vi "Configure Report Generation.vi"(8 "error in (no error)":errorcluster, 9 "Report File Path":path, 10 "Report Type":string, 11 "Execution API In":refnum<class "Execution API.lvclass">) -> (0 "error out":errorcluster, 3 "Execution API Out":refnum<class "Execution API.lvclass">)   [LabVIEW 2020, in "Execution API.lvclass"]
uses:
  Execution API.lvclass
  Plugins/Report/Report.lvclass
  C:/git/astemes-lunit/source/Framework/Plugin/Plugin.lvclass
  Execution API.lvclass/Execution API.ctl
  Plugin Loader/Plugin Loader.lvclass
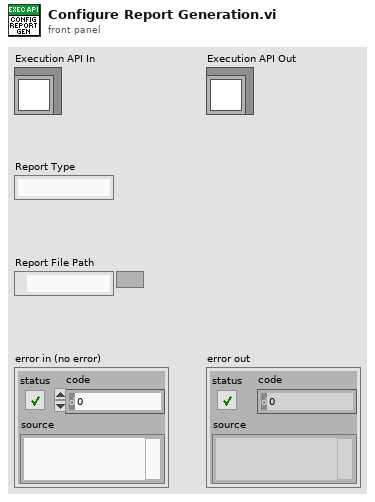
[diagram p1: front panel]
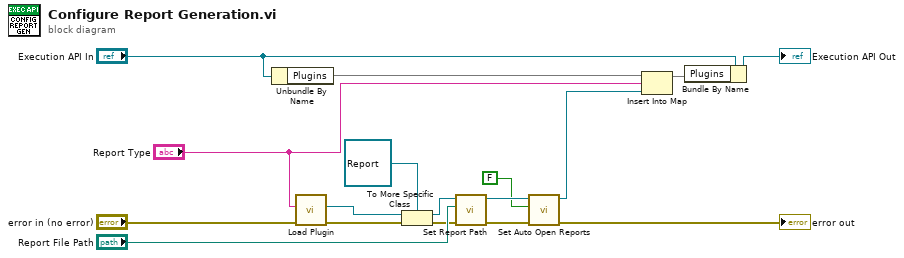
[diagram p0: block diagram]
diagram:
  n1 = Unbundle By Name("Execution API In") -> ("Plugins"=w8:map{string, refnum<class "Plugin.lvclass">})
  n2 = call "Load Plugin.vi"("error in (no error)"="error in (no error)", "Plugin"="Report Type") -> ("error out"=w11:errorcluster, "Plugin"=w14:refnum<class "Plugin.lvclass">)  [unwired: 8 in]
  n3 = To More Specific Class(target class=refnum<class "Report.lvclass"> refnum ("Report Out"), reference=w14, error in=w11) -> (specific class reference=w16:refnum<class "Report.lvclass">, error out=w13:errorcluster)
  n4 = call "Set Report Path.vi"("error in (no error)"=w13, "Report Path"="Report File Path", "Report In"=w16) -> ("error out"=w12:errorcluster, "Report Out"=w3:refnum<class "Report.lvclass">)  [unwired: 7 in]
  n5 = call "Set Auto Open Reports.vi"("error in (no error)"=w12, "Open Generated Reports?"=FALSE, "Report In"=w3) -> ("error out"=→"error out":errorcluster, "Report Out"=w2:refnum<class "Report.lvclass">)  [unwired: 7 in]
  n6 = Insert Into Map(map in=w8, key="Report Type", value=w2) -> (map out=w9:map{string, refnum<class "Plugin.lvclass">})  [unwired: 2 out]
  n7 = Bundle By Name(cluster="Execution API In", "Plugins"=w9) -> (→"Execution API Out":refnum<class "Execution API.lvclass">)
